vi "ClimbSimple.vi"() -> ()   [LabVIEW 2012]
uses:
  <vilib>/Rock Robotics/WPI/DigitalInput/WPI_DigitalInputDevRef.ctl
  <vilib>/Rock Robotics/SystemInterfaces/DIO/FPGA_DIOChannel.ctl
  <vilib>/Rock Robotics/SystemInterfaces/Typedef/FPGA_TypedefDigitalModule.ctl
  ClimbStatesSimple.ctl
  Robot Global Data.vi
panel:
  out "ResumeState":T1
  out "CommandState":T1
  in  "input cluster":T5={"ArmInOut"={"DevStatus"={"status"=FALSE, "code"=0, "source"=""}, "DIO Channel"=enum."Invalid", "Digital Module"=enum."Digital Module 1"}, "ArmMiddle"={"DevStatus"={"status"=FALSE, "code"=0, "source"=""}, "DIO Channel"=enum."Invalid", "Digital Module"=enum."Digital Module 1"}, "HooksOut"={"DevStatus"={"status"=FALSE, "code"=0, "source"=""}, "DIO Channel"=enum."Invalid", "Digital Module"=enum."Digital Module 1"}, "HooksIn"={"DevStatus"={"status"=FALSE, "code"=0, "source"=""}, "DIO Channel"=enum."Invalid", "Digital Module"=enum."Digital Module 1"}, "HooksMiddle"={"DevStatus"={"status"=FALSE, "code"=0, "source"=""}, "DIO Channel"=enum."Invalid", "Digital Module"=enum."Digital Module 1"}, "Shooter"={"DevStatus"={"status"=FALSE, "code"=0, "source"=""}, "DIO Channel"=enum."Invalid", "Digital Module"=enum."Digital Module 1"}}
  out "ArmInOut":bool
  out "ArmMiddle":bool
  out "HooksOut":bool
  out "HooksIn":bool
  out "HooksMiddle":bool
  out "Shooter":bool
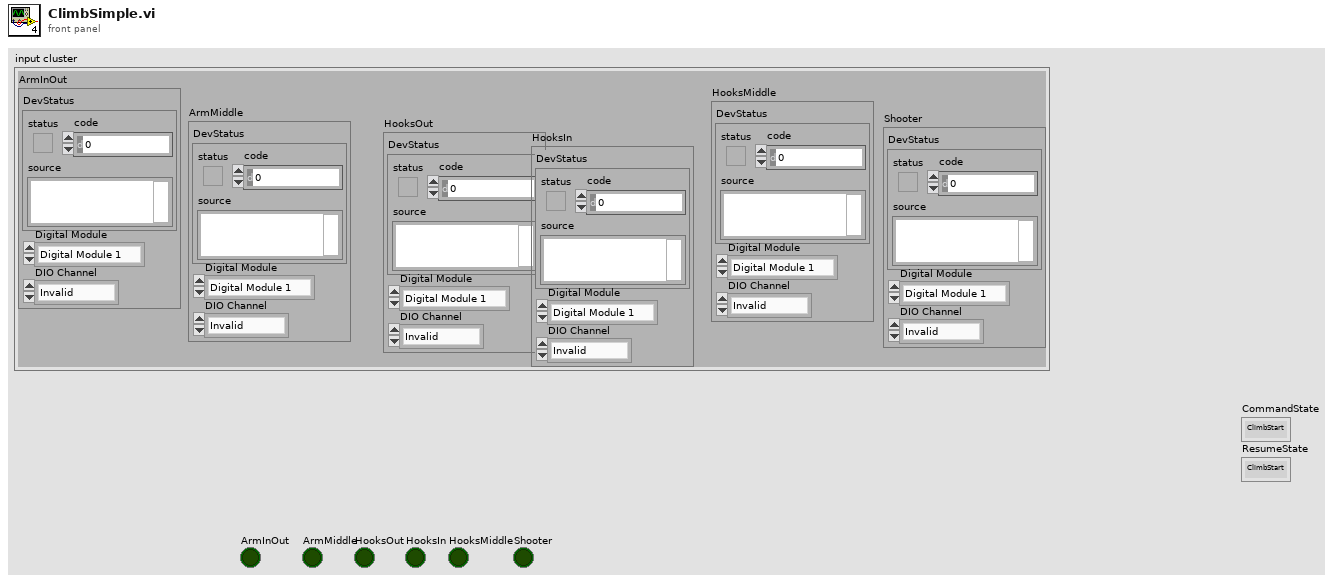
[diagram p1: front panel]
types:
  T1 = typedef "ClimbStatesSimple.ctl" = enum16{"ClimbStart", "ArmExtends", "Rachet re-engage", "Arm 60deg", "PullRobot", "Pause"}
  T2 = typedef "WPI_DigitalInputDevRef.ctl" = cluster{"DevStatus":errorcluster, "DIO Channel":T3, "Digital Module":T4}
  T3 = typedef "FPGA_DIOChannel.ctl" = enum8{"DIO 1", "DIO 2", "DIO 3", "DIO 4", "DIO 5", "DIO 6", "DIO 7", "DIO 8", "DIO 9", "DIO 10", "DIO 11", "DIO 12", "DIO 13", "DIO 14", "Invalid"}
  T4 = typedef "FPGA_TypedefDigitalModule.ctl" = enum16{"Digital Module 1", "Digital Module 2"}
  T5 = cluster{"ArmInOut":T2, "ArmMiddle":T2, "HooksOut":T2, "HooksIn":T2, "HooksMiddle":T2, "Shooter":T2}
  T6 = typedef "LoopDisable.ctl" = cluster{"Climb.vi":bool, "LauncherAngle.vi":bool, "Launcher.vi":bool, "ArmControl.vi":bool, "WinchMotor.vi":bool, "ReadDriveEncoder.vi":bool}
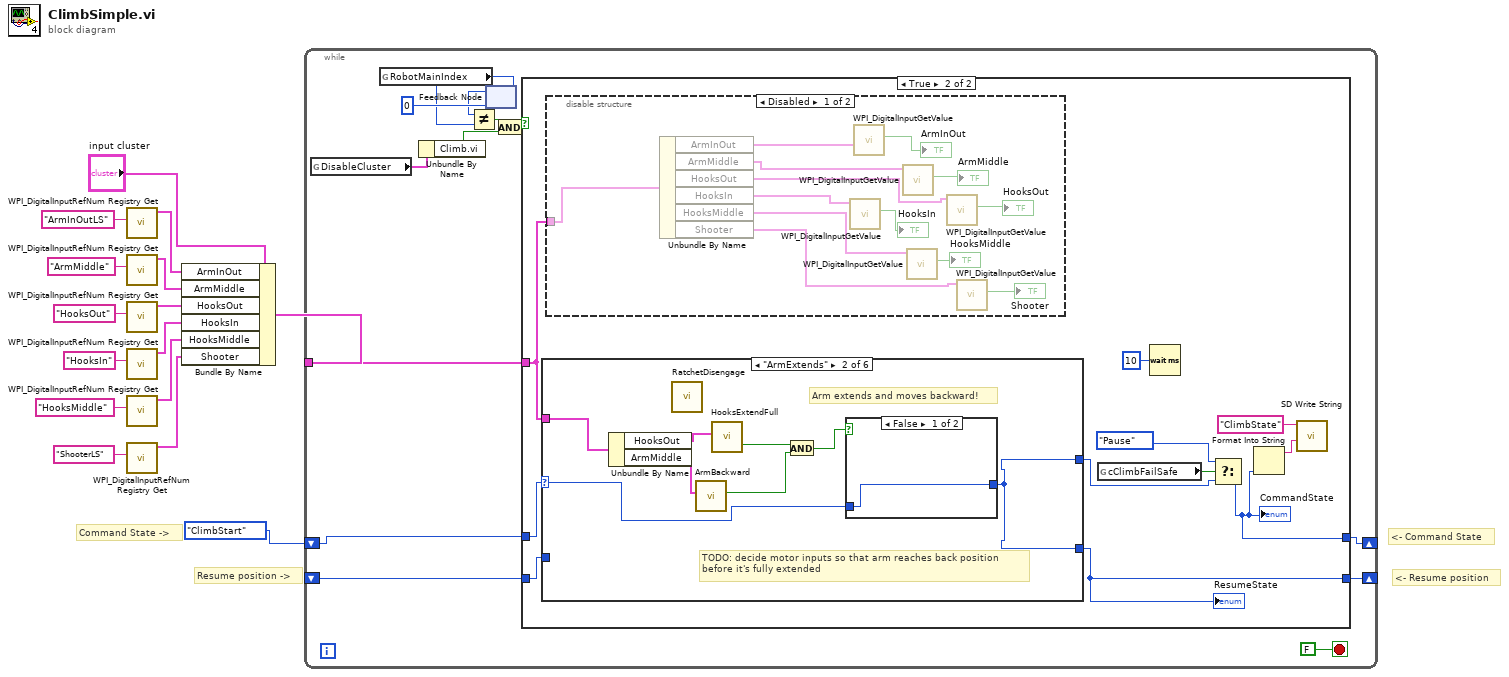
[diagram p0: block diagram]
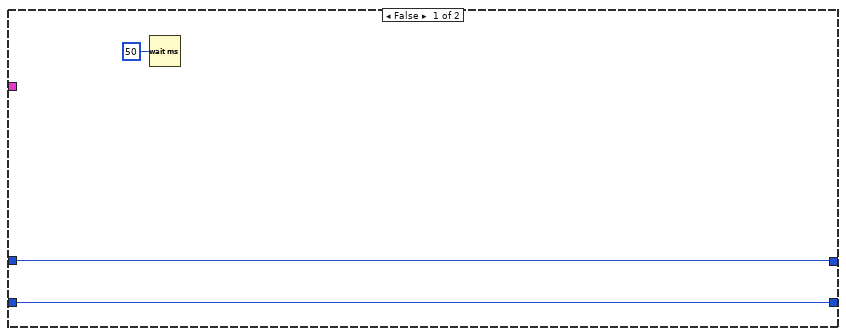
[diagram p2: hidden frame]
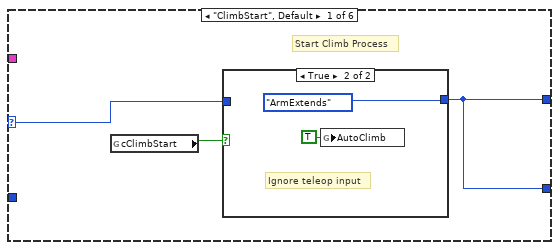
[diagram p3: hidden frame]
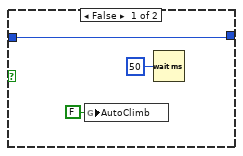
[diagram p4: hidden frame]
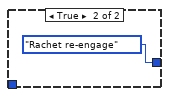
[diagram p5: hidden frame]
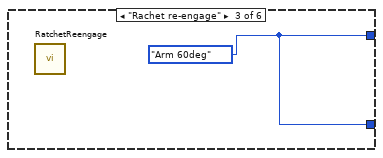
[diagram p6: hidden frame]
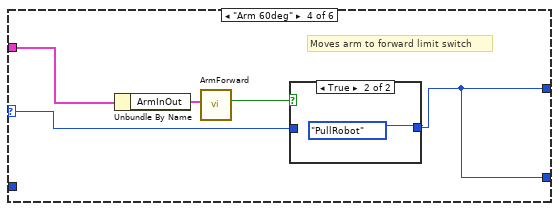
[diagram p7: hidden frame]
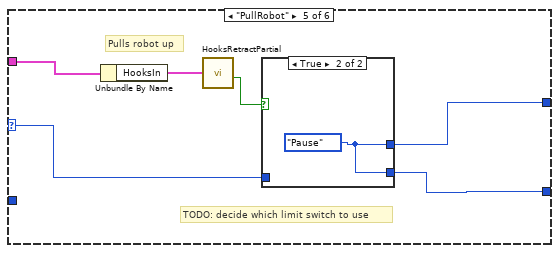
[diagram p9: hidden frame]
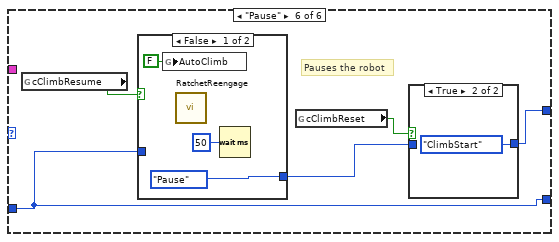
[diagram p11: hidden frame]
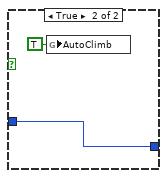
[diagram p13: hidden frame]
diagram:
  # "Resume position ->"
  # "Command State ->"
  # "<- Resume position"
  # "<- Command State"
  n1 = call <vilib>:"WPI_DigitalInputRefNum Registry Get.vi"("refnum name"="ArmInOutLS") -> ("DigitalInputDevRef"=w9:T2)  [unwired: 9 in, 1 out]
  n2 = call <vilib>:"WPI_DigitalInputRefNum Registry Get.vi"("refnum name"="ArmMiddle") -> ("DigitalInputDevRef"=w7:T2)  [unwired: 9 in, 1 out]
  n3 = call <vilib>:"WPI_DigitalInputRefNum Registry Get.vi"("refnum name"="HooksOut") -> ("DigitalInputDevRef"=w6:T2)  [unwired: 9 in, 1 out]
  n4 = call <vilib>:"WPI_DigitalInputRefNum Registry Get.vi"("refnum name"="HooksIn") -> ("DigitalInputDevRef"=w5:T2)  [unwired: 9 in, 1 out]
  n5 = call <vilib>:"WPI_DigitalInputRefNum Registry Get.vi"("refnum name"="HooksMiddle") -> ("DigitalInputDevRef"=w4:T2)  [unwired: 9 in, 1 out]
  n6 = call <vilib>:"WPI_DigitalInputRefNum Registry Get.vi"("refnum name"="ShooterLS") -> ("DigitalInputDevRef"=w3:T2)  [unwired: 9 in, 1 out]
  n7 = Bundle By Name(cluster="input cluster", "ArmInOut"=w9, "ArmMiddle"=w7, "HooksOut"=w6, "HooksIn"=w5, "HooksMiddle"=w4, "Shooter"=w3) -> (w2:T5)
  n8 = while {
    shift-right: [w26] -> _
    shift-left: _ -> [w27]
    tunnel: w2 -> [w25]
    shift-right: [w17] -> _
    shift-left: ClimbStatesSimple."ClimbStart" ("Enum") -> [w16]
    stop <- FALSE stop-if-true
    n9 = global read "Robot Global Data.vi" "DisableCluster"() -> (w18:T6)
    n10 = global read "Robot Global Data.vi" "RobotMainIndex"() -> (w23:i32)
    n11 = Unbundle By Name(w18) -> ("Climb.vi"=w19:bool)
    n12 = feedback #1(0 ("TeleopIndex")) -> (w22:i32)
    n13 = Not Equal?(x=w22, y=w23) -> (x != y?=w21:bool)
    n14 = feedback-in #1(w23) -> ()
    n15 = And(x=w21, y=w19) -> (x .and. y?=w20:bool)
    n16 = case shown="True" w20 {
      tunnel: w16 -> [w31 w37]
      tunnel: w27 -> [w30 w36]
      tunnel: [w30 w32] -> w26
      tunnel: [w31 w33] -> w17
      tunnel: w25 -> [_ w35]
      frame False {
        n17 = Wait (ms)(milliseconds to wait=u32 50) -> ()  [unwired: 1 out]
      }
      frame True {
        n18 = case shown="\"ArmExtends\"" w37 {
          selector: w37 -> [w44 w53 _ w64 w71 _]
          tunnel: w36 -> [_ _ _ _ _ w78]
          tunnel: w35 -> [_ w51 _ w63 w72 _]
          tunnel: [w43 w52 w61 w62 w69 w77] -> w34
          tunnel: [w43 w52 w61 w62 w70 w78] -> w32
          frame "ClimbStart", Default {
            # "Start Climb Process"
            n19 = global read "Robot Global Data.vi" "cClimbStart"() -> (w45:bool)
            n20 = case shown="True" w45 {
              tunnel: [w46 ClimbStatesSimple."ArmExtends" ("Enum")] -> w43
              tunnel: w44 -> [w46 _]
              frame False {
                n21 = global write "Robot Global Data.vi" "AutoClimb"(FALSE ("AutoClimb")) -> ()
                n22 = Wait (ms)(milliseconds to wait=u32 50) -> ()  [unwired: 1 out]
              }
              frame True {
                # "Ignore teleop input"
                n23 = global write "Robot Global Data.vi" "AutoClimb"(TRUE ("AutoClimb")) -> ()
              }
            }
          }
          frame "ArmExtends" {
            # "TODO: decide motor inputs so that arm reaches back position\nbefore it's fully extended"
            # "Arm extends and moves backward!"
            n24 = Unbundle By Name(w51) -> ("HooksOut"=w58:T2, "ArmMiddle"=w57:T2)
            n25 = call "RatchetDisengage.vi"() -> ()  [unwired: 12 in]
            n26 = call "ArmBackward.vi"("BackwardLimitSwitch"=w57) -> ("Done?"=w55:bool)  [unwired: 10 in]
            n27 = call "HooksExtendFull.vi"("HooksOutLimitSwitch"=w58) -> ("Done?"=w56:bool)  [unwired: 10 in]
            n28 = And(x=w56, y=w55) -> (x .and. y?=w54:bool)
            n29 = case shown="False" w54 {
              tunnel: w53 -> [w59 _]
              tunnel: [w59 ClimbStatesSimple."Rachet re-engage" ("Enum")] -> w52
              frame False {
              }
              frame True {
              }
            }
          }
          frame "Rachet re-engage" {
            w61 = ClimbStatesSimple."Arm 60deg" ("Enum")
            n30 = call "RatchetReengage.vi"() -> ()  [unwired: 12 in]
          }
          frame "Arm 60deg" {
            # "Moves arm to forward limit switch"
            n31 = Unbundle By Name(w63) -> ("ArmInOut"=w66:T2)
            n32 = call "ArmForward.vi"("ForwardLimitSwitch"=w66) -> ("Done?"=w65:bool)  [unwired: 10 in]
            n33 = case shown="True" w65 {
              tunnel: w64 -> [w67 _]
              tunnel: [w67 ClimbStatesSimple."PullRobot" ("Enum")] -> w62
              frame False {
              }
              frame True {
              }
            }
          }
          frame "PullRobot" {
            # "TODO: decide which limit switch to use"
            # "Pulls robot up"
            n34 = Unbundle By Name(w72) -> ("HooksIn"=w74:T2)
            n35 = call "HooksRetractPartial.vi"("HooksMiddleLimitSwitch"=w74) -> ("Done?"=w73:bool)  [unwired: 10 in]
            n36 = case shown="True" w73 {
              tunnel: w71 -> [w75 _]
              tunnel: [w75 w76] -> w70
              tunnel: [w75 w76] -> w69
              frame False {
              }
              frame True {
                w76 = ClimbStatesSimple."Pause" ("Enum")
              }
            }
          }
          frame "Pause" {
            # "Pauses the robot"
            n37 = global read "Robot Global Data.vi" "cClimbResume"() -> (w81:bool)
            n38 = case shown="False" w81 {
              tunnel: w78 -> [_ w88]
              tunnel: [ClimbStatesSimple."Pause" ("Enum") w88] -> w79
              frame False {
                n39 = global write "Robot Global Data.vi" "AutoClimb"(FALSE ("AutoClimb")) -> ()
                n40 = call "RatchetReengage.vi"() -> ()  [unwired: 12 in]
                n41 = Wait (ms)(milliseconds to wait=u32 50) -> ()  [unwired: 1 out]
              }
              frame True {
                n42 = global write "Robot Global Data.vi" "AutoClimb"(TRUE ("AutoClimb")) -> ()
              }
            }
            n43 = global read "Robot Global Data.vi" "cClimbReset"() -> (w80:bool)
            n44 = case shown="True" w80 {
              tunnel: [w82 ClimbStatesSimple."ClimbStart" ("Enum")] -> w77
              tunnel: w79 -> [w82 _]
              frame False {
              }
              frame True {
              }
            }
          }
        }
        "ResumeState" <- w32
        n45 = disable-structure shown="Disabled" {
          disable-tunnel: w35 -> [w101 _]
          frame Disabled {
            n46 = Unbundle By Name(w101) -> ("ArmInOut"=w100:T2, "ArmMiddle"=w98:T2, "HooksOut"=w96:T2, "HooksIn"=w94:T2, "HooksMiddle"=w92:T2, "Shooter"=w90:T2)
            n47 = call <vilib>:"WPI_DigitalInputGetValue.vi"("DigitalInputDevRef"=w94) -> ("Value"=→"HooksIn":bool)  [unwired: 8 in, 2 out]
            n48 = call <vilib>:"WPI_DigitalInputGetValue.vi"("DigitalInputDevRef"=w100) -> ("Value"=→"ArmInOut":bool)  [unwired: 8 in, 2 out]
            n49 = call <vilib>:"WPI_DigitalInputGetValue.vi"("DigitalInputDevRef"=w98) -> ("Value"=→"ArmMiddle":bool)  [unwired: 8 in, 2 out]
            n50 = call <vilib>:"WPI_DigitalInputGetValue.vi"("DigitalInputDevRef"=w92) -> ("Value"=→"HooksMiddle":bool)  [unwired: 8 in, 2 out]
            n51 = call <vilib>:"WPI_DigitalInputGetValue.vi"("DigitalInputDevRef"=w96) -> ("Value"=→"HooksOut":bool)  [unwired: 8 in, 2 out]
            n52 = call <vilib>:"WPI_DigitalInputGetValue.vi"("DigitalInputDevRef"=w90) -> ("Value"=→"Shooter":bool)  [unwired: 8 in, 2 out]
          }
          frame Enabled {
          }
        }
        n53 = global read "Robot Global Data.vi" "cClimbFailSafe"() -> (w42:bool)
        n54 = Wait (ms)(milliseconds to wait=u32 10) -> ()  [unwired: 1 out]
        n55 = Select(t=ClimbStatesSimple."Pause" ("Enum"), s=w42, f=w34) -> (s? t:f=w33:T1)
        "CommandState" <- w33
        n56 = Format Into String(w33) -> (resulting string=w40:string)  [unwired: 3 in, 1 out]
        n57 = call <vilib>:"SD Write String.vi"("String"=w40, "Name"="ClimbState") -> ()  [unwired: 8 in, 2 out]
      }
    }
  }
